vi "getRandomVideos.vi"(8 "error in (no error)":errorcluster) -> (0 "error out":errorcluster, 3 "HashMap":T1)   [LabVIEW 2018, in "ThirdPartyYoutubeClass.lvclass"]
uses:
  ThirdPartyYoutubeClass.lvclass
  Globals/HashMap.ctl
  Video Class/Video.lvclass
  ConsoleOut/Print Options.ctl
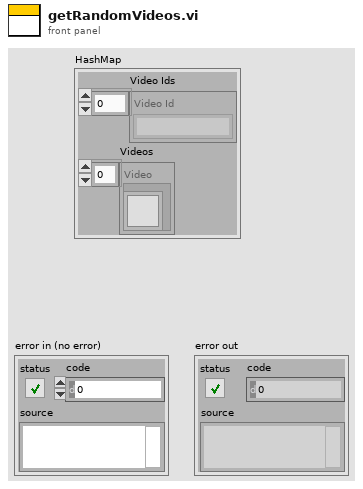
[diagram p1: front panel]
types:
  T1 = typedef "HashMap.ctl" = cluster{"Video Ids":string[], "Videos":refnum<class "Video.lvclass">[]}
  T2 = typedef "Print Options.ctl" = enum16{"Create", "Get Reference", "Print", "Print Header", "Close"}
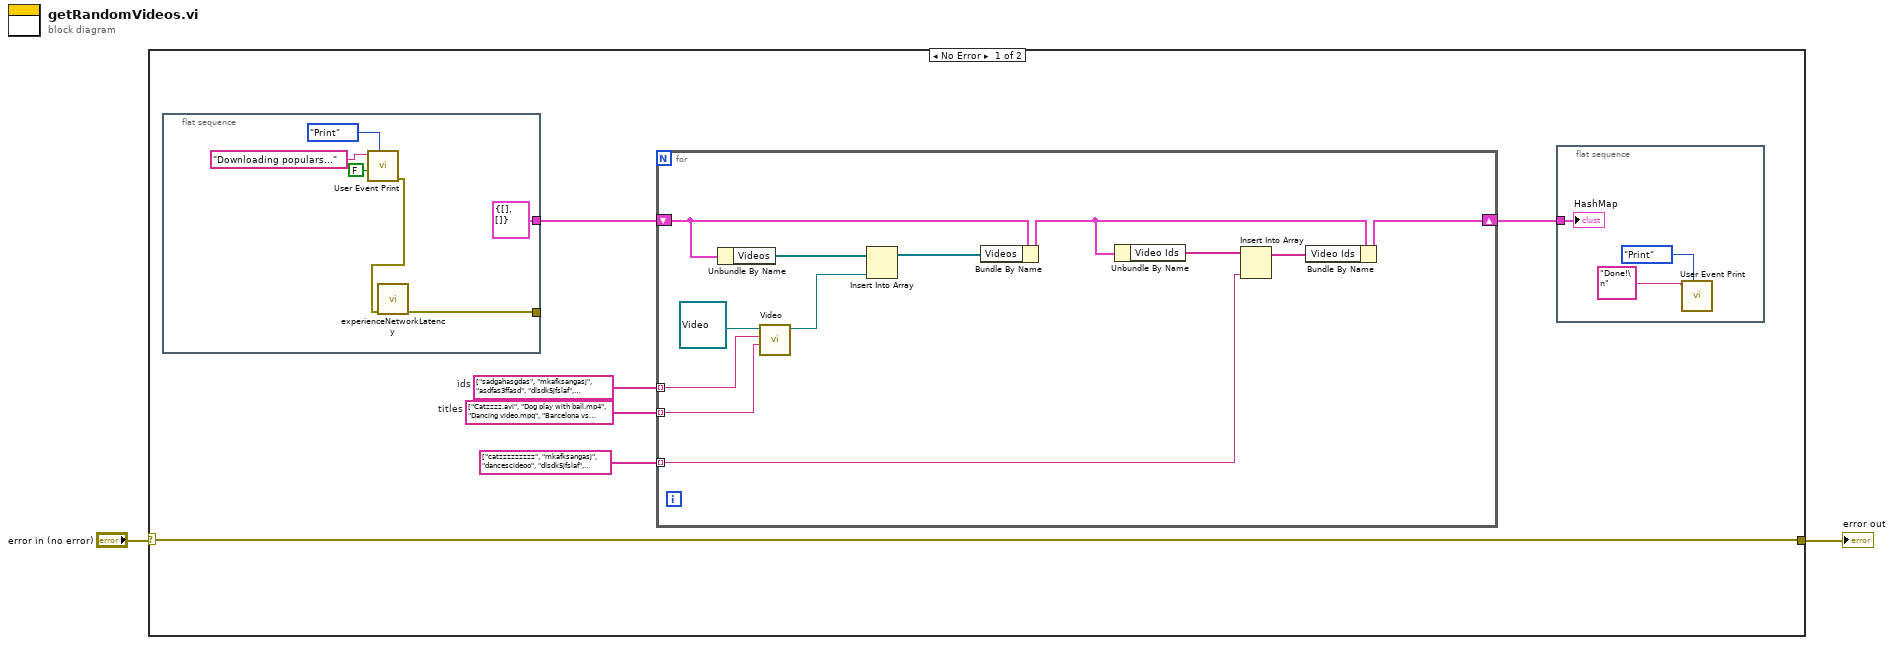
[diagram p0: block diagram]
diagram:
  n1 = case shown="No Error" "error in (no error)" {
    selector: "error in (no error)" -> [w3 w30]
    tunnel: [w3 w30] -> w1
    frame No Error {
      w6 = string[] ["Catzzzz.avi", "Dog play with ball.mp4", "Dancing video.mpq", "Barcelona vs RealM.mov", "Programing lesson#1.avi"]  # titles
      w7 = string[] ["sadgahasgdas", "mkafksangasj", "asdfas3ffasd", "dlsdk5jfslaf", "3sdfgsd1j333"]  # ids
      n2 = flat-sequence {
        tunnel: [w29] -> _
        tunnel: [T1 {"Video Ids"=[], "Videos"=[]} ("HashMap")] -> w8
        frame #0 {
          n3 = call "User Event Print.vi"("Options"=Print_Options."Print", "add EOL? (T)"=FALSE, "String to Print"="Downloading populars..." ("ConsoleOut")) -> ("error out"=w26:errorcluster)  [unwired: 7 in, 1 out]
          n4 = call "experienceNetworkLatency.vi"("error in (no error)"=w26) -> ("error out"=w29:errorcluster)  [unwired: 10 in]
        }
      }
      n5 = for {
        shift-right: [w15] -> w4
        shift-left: w8 -> [w23]
        tunnel: w7 -> [w18] mode=indexing
        tunnel: w6 -> [w17] mode=indexing
        tunnel: string[] ["catzzzzzzzzz", "mkafksangasj", "dancescideoo", "dlsdk5jfslaf", "3sdfgsd1j333"] -> [w12] mode=indexing
        n6 = Unbundle By Name(w23) -> ("Videos"=w22:refnum<class "Video.lvclass">[])
        n7 = call "Video.vi"("title"=w17, "id"=w18, "Video in"=refnum<class "Video.lvclass"> refnum ("Video.lvclass")) -> ("Video out"=w19:refnum<class "Video.lvclass">)  [unwired: 7 in, 1 out]
        n8 = Insert Into Array(array=w22, new element=w19) -> (w21:refnum<class "Video.lvclass">[])  [unwired: 1 in]
        n9 = Bundle By Name(cluster=w23, "Videos"=w21) -> (w16:T1)
        n10 = Unbundle By Name(w16) -> ("Video Ids"=w14:string[])
        n11 = Insert Into Array(array=w14, new element=w12) -> (w13:string[])  [unwired: 1 in]
        n12 = Bundle By Name(cluster=w16, "Video Ids"=w13) -> (w15:T1)
      }
      n13 = flat-sequence {
        tunnel: w4 -> [w11]
        frame #0 {
          n14 = call "User Event Print.vi"("Options"=Print_Options."Print", "String to Print"="Done!\n" ("ConsoleOut")) -> ()  [unwired: 8 in, 2 out]
          "HashMap" <- w11
        }
      }
    }
    frame Error {
    }
  }
  "error out" <- w1
